vi "Scope String.vi"(11 "Get Library Access Scope":T1(ring)) -> (3 "String":string)   [LabVIEW 2023, in "VIDoc Printer.lvlib" / "VIDoc Printer.lvclass"]
doc: "Converts the Access Scope into a printable String"
uses:
  VIDoc Printer.lvclass
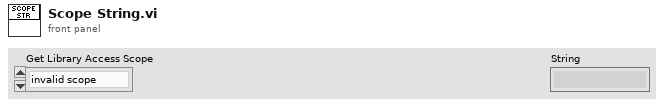
[diagram p1: front panel]
types:
  T1 = enum32{"invalid scope", "public", "private", "protected", "community"}
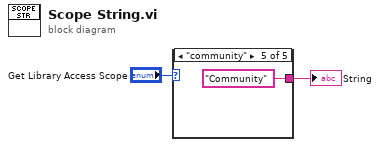
[diagram p0: block diagram]
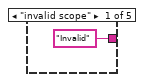
[diagram p2: hidden frame]
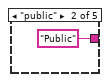
[diagram p3: hidden frame]
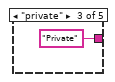
[diagram p4: hidden frame]
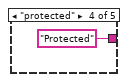
[diagram p5: hidden frame]
diagram:
  n1 = case shown="\"community\"" "Get Library Access Scope" {
    tunnel: ["Invalid" "Public" "Private" "Protected" "Community"] -> w1
    frame "invalid scope" {
    }
    frame "public" {
    }
    frame "private" {
    }
    frame "protected" {
    }
    frame "community" {
    }
  }
  "String" <- w1
